vi "text_test.vi"() -> ()   [LabVIEW 2010]
panel:
  in  "Path":path
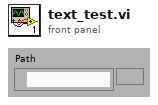
[diagram p1: front panel]
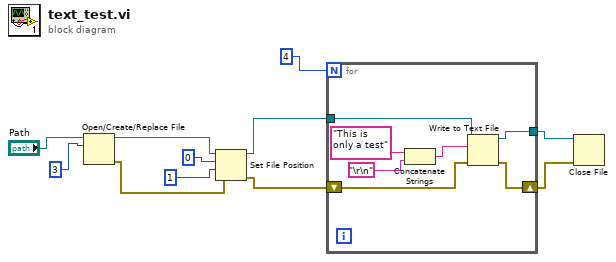
[diagram p0: block diagram]
diagram:
  n1 = Open/Create/Replace File(file path (use dialog)="Path", operation (0:open)=3) -> (refnum out=w6:refnum<file>, error out=w4:errorcluster)  [unwired: 4 in, 1 out]
  n2 = Set File Position(offset (in bytes) (0)=0, refnum=w6, from (0:start)=1, error in=w4) -> (refnum out=w5:refnum<file>, error out=w3:errorcluster)
  n3 = for {
    N: 4 -> [_]
    tunnel: w5 -> [w18]
    tunnel: [w17] -> w9
    shift-right: [w15] -> w8
    shift-left: w3 -> [w16]
    n4 = Concatenate Strings("This is only a test", "\r\n") -> (w12:string)
    n5 = Write to Text File(file (use dialog)=w18, text=w12, error in=w16) -> (refnum out=w17:refnum<file>, error out=w15:errorcluster)  [unwired: 1 in, 1 out]
  }
  n6 = Close File(refnum=w9, error in=w8) -> ()  [unwired: 2 out]
